vi "Write Test Information to TDMS.vi"(6 "Test No.":i32, 8 "error in (no error)":errorcluster, 9 "Test Information":T1, 10 "Test Sequence":T2 {"Total Test Energy (J)" format="%#_4p"}, 11 "Refnum in":refnum<k34>) -> (0 "error out":errorcluster, 3 "Refnum out":refnum<k34>)   [LabVIEW 2015]
doc: "Writes the Test Sequence and Test Information clusters to the TDMS Group Description."
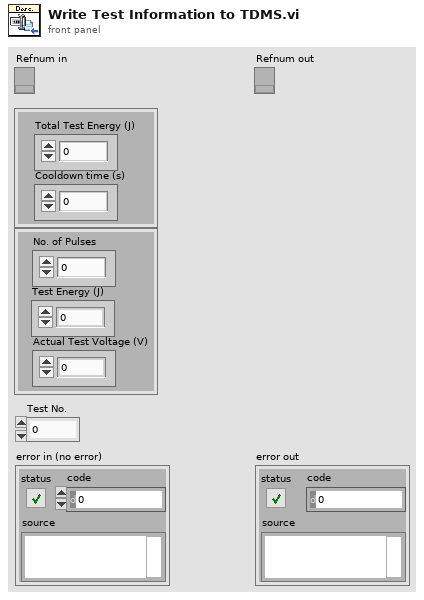
[diagram p1: front panel]
types:
  T1 = cluster{"No. of Pulses":i32, "Test Energy (J)":dbl, "Actual Test Voltage (V)":dbl}
  T2 = cluster{"Cooldown time (s)":dbl, "Total Test Energy (J)":dbl}
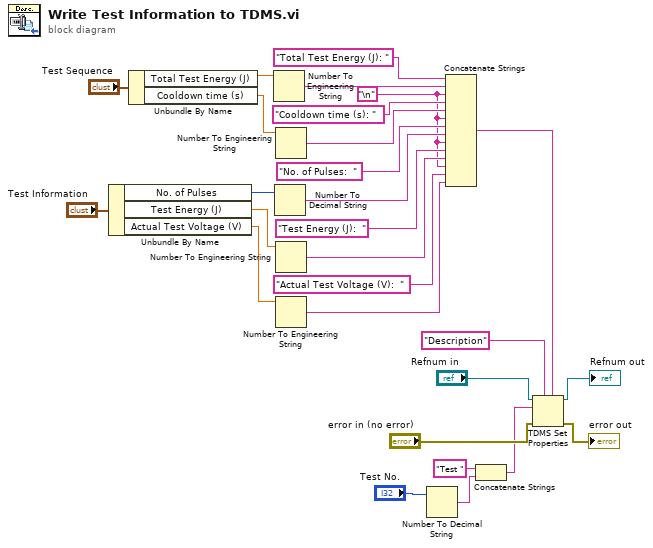
[diagram p0: block diagram]
diagram:
  w4 = "\n"
  n1 = Unbundle By Name("Test Information") -> ("No. of Pulses"=w11:i32, "Test Energy (J)"=w10:dbl, "Actual Test Voltage (V)"=w9:dbl)
  n2 = Unbundle By Name("Test Sequence") -> ("Total Test Energy (J)"=w16:dbl, "Cooldown time (s)"=w14:dbl)
  n3 = Number To Engineering String(4:w16) -> (0:w15:string)  [unwired: 3 in]
  n4 = Number To Decimal String(number=w11) -> (decimal integer string=w7:string)  [unwired: 1 in]
  n5 = Number To Engineering String(4:w14) -> (0:w13:string)  [unwired: 3 in]
  n6 = Number To Engineering String(4:w10) -> (0:w5:string)  [unwired: 3 in]
  n7 = Number To Engineering String(4:w9) -> (0:w2:string)  [unwired: 3 in]
  n8 = Number To Decimal String(number="Test No.") -> (decimal integer string=w23:string)  [unwired: 1 in]
  n9 = Concatenate Strings("Total Test Energy (J): " ("string"), w15, w4, "Cooldown time (s): " ("string"), w13, w4, "No. of Pulses:  " ("string"), w7, w4, "Test Energy (J):  " ("string"), w5, w4, "Actual Test Voltage (V):  " ("string"), w2) -> (w1:string)
  n10 = Concatenate Strings("Test " ("string"), w23) -> (w20:string)
  n11 = TDMS Set Properties(5:w1, 7:"Description", 8:"error in (no error)", 10:w20, 11:"Refnum in") -> (0:→"error out":errorcluster, 3:→"Refnum out":refnum<k34>)  [unwired: 1 in, 2 out]
